vi "PositionToHub.vi"(4 "Position":dbl[](array[numeric])) -> (1 "位置簇":cluster{"控制电机":T1, "位置":dbl}[](array[cluster]))   [LabVIEW 2018]
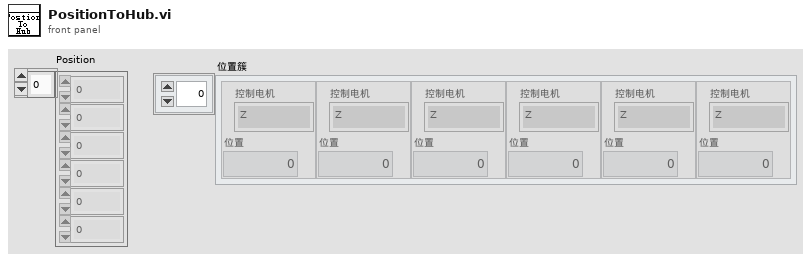
[diagram p1: front panel]
types:
  T1 = typedef "控制电机枚举器.ctl" = enum16{"Z", "Y", "X", "发散角", "俯仰", "旋转"}
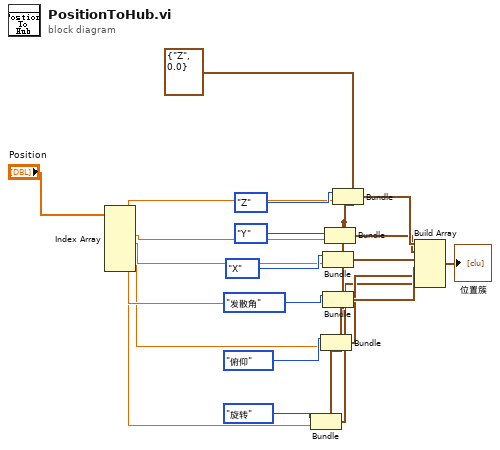
[diagram p0: block diagram]
diagram:
  w8 = cluster{"控制电机":T1, "位置":dbl} {"控制电机"=enum."Z", "位置"=0.0} ("元素")
  n1 = Index Array(array="Position") -> (element #1=w19:dbl, element #2=w17:dbl, element #3=w15:dbl, element #4=w13:dbl, element #5=w11:dbl, element #6=w9:dbl)  [unwired: 6 in]
  n2 = Bundle(cluster=w8, "控制电机"=控制电机枚举器."旋转", "位置"=w9) -> (w2:cluster{"控制电机":T1, "位置":dbl})
  n3 = Bundle(cluster=w8, "控制电机"=控制电机枚举器."俯仰", "位置"=w11) -> (w3:cluster{"控制电机":T1, "位置":dbl})
  n4 = Bundle(cluster=w8, "控制电机"=控制电机枚举器."X", "位置"=w15) -> (w5:cluster{"控制电机":T1, "位置":dbl})
  n5 = Bundle(cluster=w8, "控制电机"=控制电机枚举器."发散角", "位置"=w13) -> (w4:cluster{"控制电机":T1, "位置":dbl})
  n6 = Bundle(cluster=w8, "控制电机"=控制电机枚举器."Y", "位置"=w17) -> (w6:cluster{"控制电机":T1, "位置":dbl})
  n7 = Bundle(cluster=w8, "控制电机"=控制电机枚举器."Z", "位置"=w19) -> (w7:cluster{"控制电机":T1, "位置":dbl})
  n8 = Build Array(w7, w6, w5, w4, w3, w2) -> (→"位置簇":cluster{"控制电机":T1, "位置":dbl}[])
